vi "Advanced Remez FIR Filter Design.vi"() -> ()   [LabVIEW 2023]
doc: "Demonstrates how to use the DFD Remez Design VI to design advanced finite impulse response (FIR) filters. You can learn how to configure the controls to obtain the ideal filter frequency response of the filter you want to design.\n\nComplete the following steps to use this VI.\n1) Run the VI.\n2) Select one example filter in the <B>Examples</B> list. This VI provides pre-defined filter specifications for each example filter. \n3) View the <B>Specifications</B> page to study the corresponding settings that describe the ideal frequency response.\n4) Observe the plots on the Magnitude Response, Phase Response, and Pole-Zero Plot graphs to see the characteristics of the designed filter.\n5) Compare the <B>Actual Ripples</B> listed on the <B>Magnitude Response</B> page with the <B>ripple constraint</B> specification of each frequency band. Verify if the actual ripples are less than the pre-defined settings.\n6) Click the <B>STOP</B> button to stop this VI."
uses:
  <vilib>/addons/Digital Filter Design/_REMEZ.llb/remez_fir filter type.ctl
  <vilib>/addons/Digital Filter Design/_Objects.llb/DFD Adv Band Spec.ctl
  <vilib>/addons/Digital Filter Design/_Objects.llb/DFD Phase Setting.ctl
  <vilib>/addons/Digital Filter Design/_Objects.llb/DFD Filter Obj.ctl
  <vilib>/addons/Digital Filter Design/_Objects.llb/DFD Filter Coef.ctl
  <vilib>/addons/Digital Filter Design/_Objects.llb/DFD Filter Structure Type Selector.ctl
  <vilib>/addons/Digital Filter Design/_Objects.llb/dfd_Internal Quantization Settings.ctl
  <vilib>/addons/Digital Filter Design/_Objects.llb/dfd_Internal Quantization Srcs.ctl
  <vilib>/addons/Digital Filter Design/_Objects.llb/DFD Coef Norm Type.ctl
  <vilib>/addons/Digital Filter Design/_Objects.llb/DFD Pole-Zero Plot.ctl
  <vilib>/addons/Digital Filter Design/Analysis.llb/DFD Plot Freq Response (Linear-Spaced).vi
  <vilib>/addons/Digital Filter Design/NI_DigFilterLicensed.lvlib
panel:
  in  "filter out":T1={"mSRate_Fs"=1.0, "mSRate_Version"="1.0", "mSRate_Comments"="", "mSRate_OrgCoef"={"type"=enum."Undefined", "gain"=1.0, "coef a (k)"=[], "coef b (v)"=[]}, "mSRate_CurCoef"={"type"=enum."Undefined", "gain"=1.0, "coef a (k)"=[], "coef b (v)"=[]}, "mSRate_Quantized?"=FALSE, "mSRate_QCoef"={"type"=enum."Undefined", "gain"=1.0, "coef a (k)"=[], "coef b (v)"=[]}, "mSRate_QSettings"=[], "mSRate_Order"=0, "mSRate_Scaling"={"mSRate_ScaleByPowerOf2?"=FALSE, "mSRate_ScaleType"=enum."No Norm"}} {"mSRate_QSettings"."source" items=["Coef a/k"=0, "Coef b/v"=7, "Input"=1, "Output"=2, "Multiplicand"=3, "Product"=4, "Sum"=5, "Delay"=6, "Gain"=8]}
  out "Status Str":string="Idle"
  out "Status LED":bool
  in  "Graph":T7(tab)
  out "Actual Ripples":dbl[](array[numeric])
  in  "dB On?":bool
  out "Magnitude Response":cluster{"f0":dbl, "df":dbl, "values":dbl[]}[](graph)
  in  "phase view":T8={"unwrap? (F)"=TRUE, "degree? (F)"=FALSE}
  out "Phase Response":cluster{"f0":dbl, "df":dbl, "values":dbl[]}[](graph)
  out "Z-Plane":T9
  out "Actual Order":i32
  in  "stop":bool
  in  "Selector":enum32{"Examples", "Specifications"}(tab)
  out "Description":string
  in  "Example List":i32(listbox)
  in  "Apply":bool
  in  "Frequencies of Exact Gain [Hz]":dbl[](array[numeric])
  in  "Minimum Order":enum32{"User Defined", "MinEven", "MinOdd"}(ring)
  in  "Band Specifications":T10[](array[typedef])=[{"band specification"=[{"freq"=0.0, "amplitude"=0.0, "weight"=2.0}, {"freq"=0.2, "amplitude"=0.0, "weight"=2.0}], "ripple constraint"=0.0}, {"band specification"=[{"freq"=0.25, "amplitude"=1.0, "weight"=1.0}, {"freq"=0.5, "amplitude"=1.0, "weight"=1.0}], "ripple constraint"=0.0}]
  in  "Sampling Frequency [Hz]":dbl=1.0 format="%.2f"
  in  "Filter Order":i32=52
  in  "Filter Type":T11
  # "Select Help>>Show Context Help and move the cursor over the VI icon for more information."
  # "freq"
  # "amplitude"
  # "weight"
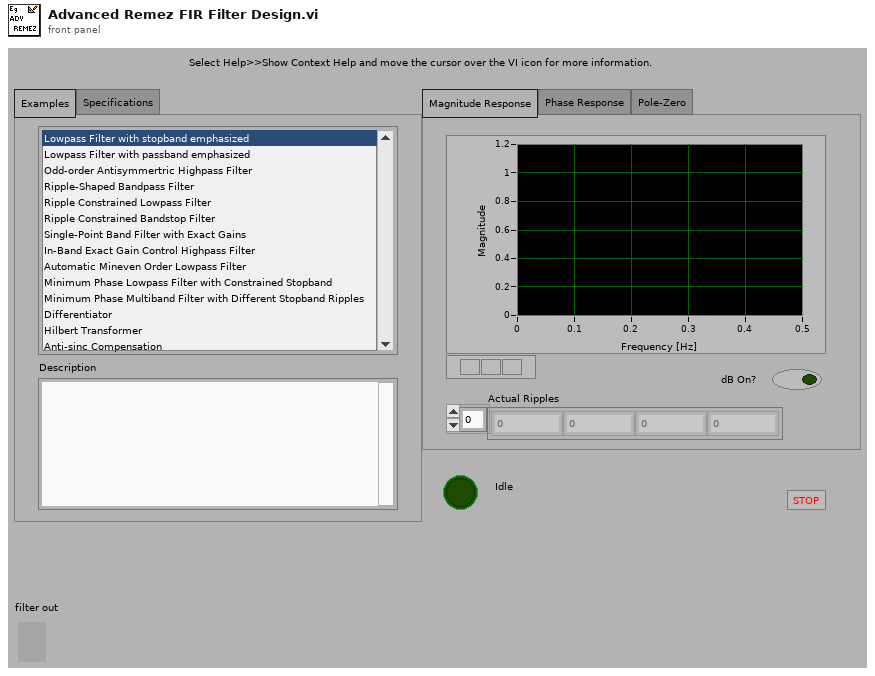
[diagram p1: front panel]
types:
  T1 = typedef "NI_DigFilterLicensed.lvlib/DFD Filter Obj.ctl" = cluster{"mSRate_Fs":dbl, "mSRate_Version":string, "mSRate_Comments":string, "mSRate_OrgCoef":T2, "mSRate_CurCoef":T2, "mSRate_Quantized?":bool, "mSRate_QCoef":T2, "mSRate_QSettings":T4[], "mSRate_Order":i32, "mSRate_Scaling":cluster{"mSRate_ScaleByPowerOf2?":bool, "mSRate_ScaleType":T6}}
  T2 = typedef "NI_DigFilterLicensed.lvlib/DFD Filter Coef.ctl" = cluster{"type":T3, "gain":dbl, "coef a (k)":dbl[], "coef b (v)":dbl[]}
  T3 = typedef "NI_DigFilterLicensed.lvlib/DFD Filter Structure Type Selector.ctl" = enum16{"Undefined", "FIR Direct Form", "FIR Direct Form Transposed", "FIR Symmetric", "FIR Antisymmetric", "IIR Direct Form I", "IIR Direct Form I Transposed", "IIR Direct Form II", "IIR Direct Form II Transposed", "IIR Cascaded Second Order Sections Form I", "IIR Cascaded Second Order Sections Form I Transposed", "IIR Cascaded Second Order Sections Form II", "IIR Cascaded Second Order Sections Form II Transposed", "Lattice Allpass (basic sections)", "Lattice Allpass (one multiplier sections)", "Lattice Allpass (normalized sections)", "Lattice AR (basic sections)", "Lattice AR (one multiplier sections)", "Lattice AR (normalized sections)", "Lattice MA (minimum phase)", "Lattice MA (maximum phase)", "Lattice ARMA (basic sections)", "Lattice ARMA (one multiplier sections)", "Lattice ARMA (normalized sections)"}
  T4 = typedef "NI_DigFilterLicensed.lvlib/dfd_Internal Quantization Settings.ctl" = cluster{"source":T5, "wl":i16, "iwl":i16, "overflow mode":enum16{"Saturation", "Wrap"}, "rounding mode":enum16{"Nearest", "Truncation"}, "signed?":bool}
  T5 = typedef "NI_DigFilterLicensed.lvlib/dfd_Internal Quantization Srcs.ctl" = u16
  T6 = typedef "NI_DigFilterLicensed.lvlib/DFD Coef Norm Type.ctl" = enum16{"No Norm", "Time Domain 1-Norm", "Time Domain 2-Norm", "Time Domain Inf-Norm"}
  T7 = enum32{"Magnitude Response", "Phase Response", "Pole-Zero"}
  T8 = typedef "NI_DigFilterLicensed.lvlib/DFD Phase Setting.ctl" = cluster{"unwrap? (F)":bool, "degree? (F)":bool}
  T9 = typedef "NI_DigFilterLicensed.lvlib/DFD Pole-Zero Plot.ctl" = cluster{dbl[], dbl[]}[]
  T10 = typedef "NI_DigFilterLicensed.lvlib/DFD Adv Band Spec.ctl" = cluster{"band specification":cluster{"freq":dbl, "amplitude":dbl, "weight":dbl}[], "ripple constraint":dbl}
  T11 = typedef "NI_DigFilterLicensed.lvlib/remez_fir filter type.ctl" = enum32{"Symmetric", "Antisymmetric", "Differentiator", "Hilbert", "Minimum Phase", "Maximum Phase"}
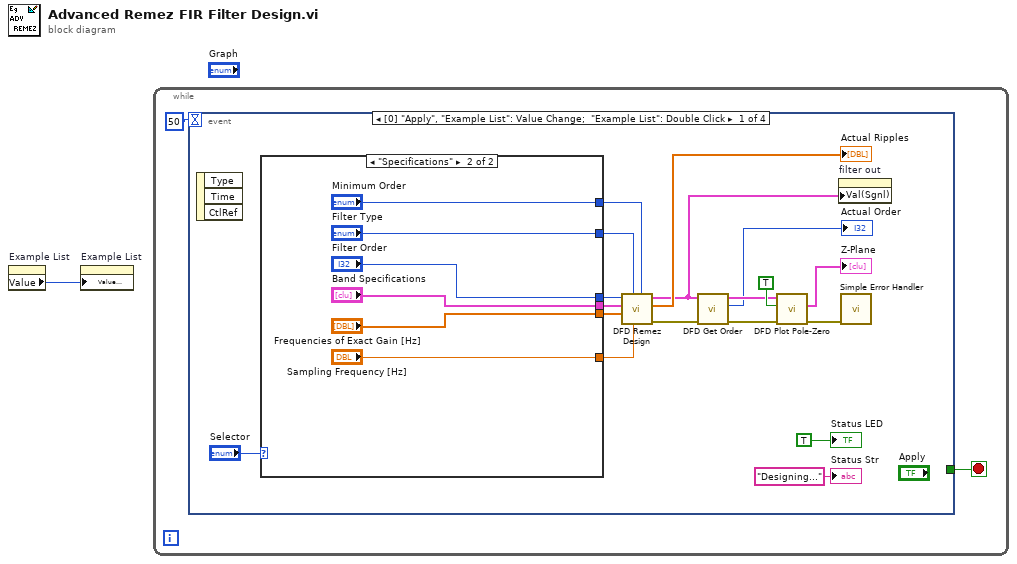
[diagram p0: block diagram]
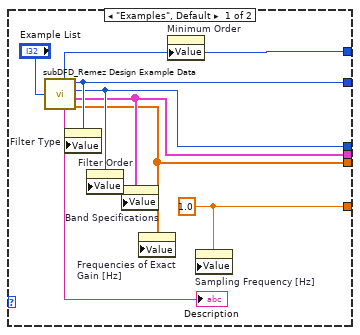
[diagram p2: hidden frame]
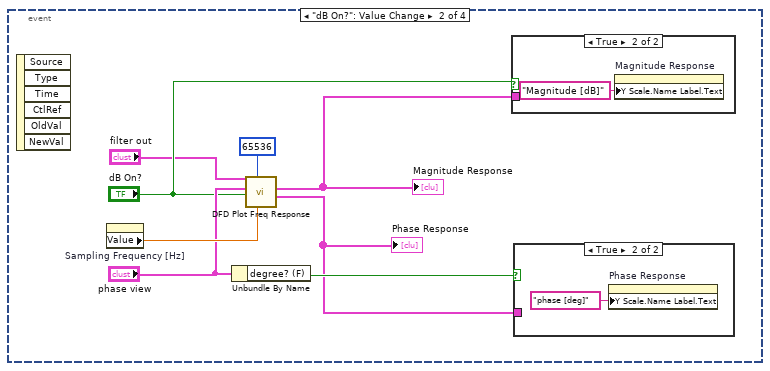
[diagram p3: hidden frame]
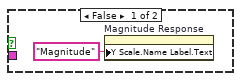
[diagram p4: hidden frame]
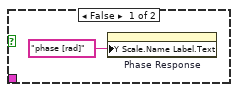
[diagram p5: hidden frame]
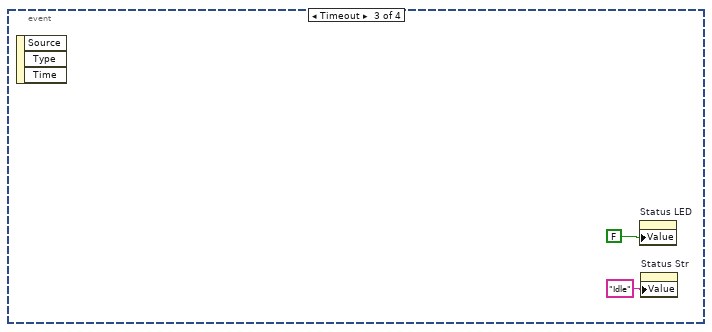
[diagram p6: hidden frame]
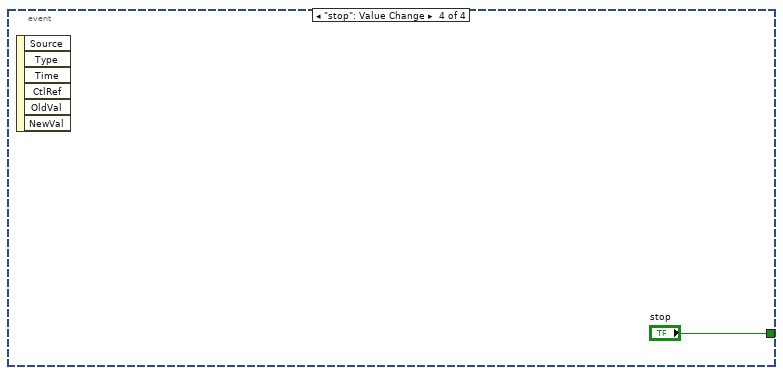
[diagram p7: hidden frame]
diagram:
  n1 = property on="Example List" class="LstBox (strict)"() -> ("Value"=w1:i32)  [unwired: 2 in, 2 out]
  n2 = property on="Example List" class="LstBox (strict)"("Value (Signaling)"=w1) -> ()  [unwired: 2 in, 2 out]
  n3 = while {
    stop <- w3 stop-if-true
    n4 = event shown="[0] \"Apply\", \"Example List\": Value Change;  \"Example List\": Double Click" {
      selector: _ -> [_ _ _ _]
      dyn-events: _ -> [_ _ _ _]
      timeout: 50 -> [_ _ _ _]
      tunnel: [_ _ _ "stop"] -> w3
      event "Apply", "Example List": Value Change; "Example List": Double Click {
        n5 = event-data() -> ()  [unwired: 4 out]
        n6 = case shown="\"Specifications\"" "Selector" {
          tunnel: [w28 "Minimum Order"] -> w18
          tunnel: [w27 "Filter Type"] -> w17
          tunnel: [w26 "Filter Order"] -> w16
          tunnel: [w25 "Band Specifications"] -> w15
          tunnel: [w24 "Frequencies of Exact Gain [Hz]"] -> w14
          tunnel: [w23 "Sampling Frequency [Hz]"] -> w13
          frame "Examples", Default {
            w23 = 1.0 ("fs [Hz]")
            n7 = call "subDFD_Remez Design Example Data.vi"("Example Idx"="Example List") -> ("minimum order"=w28:enum32{"User Defined", "MinEven", "MinOdd"}, "description"=→"Description":string, "phase option"=w27:T11, "order"=w26:i32, "band specs"=w25:T10[], "freqs of exact gain"=w24:dbl[])
            n8 = property on="Filter Type" class="Enum (strict)"("Value"=w27) -> ()  [unwired: 2 in, 2 out]
            n9 = property on="Filter Order" class="DigNum (strict)"("Value"=w26) -> ()  [unwired: 2 in, 2 out]
            n10 = property on="Band Specifications" class="Arr (strict)"("Value"=w25) -> ()  [unwired: 2 in, 2 out]
            n11 = property on="Frequencies of Exact Gain [Hz]" class="Arr (strict)"("Value"=w24) -> ()  [unwired: 2 in, 2 out]
            n12 = property on="Minimum Order" class="Enum (strict)"("Value"=w28) -> ()  [unwired: 2 in, 2 out]
            n13 = property on="Sampling Frequency [Hz]" class="DigNum (strict)"("Value"=w23) -> ()  [unwired: 2 in, 2 out]
          }
          frame "Specifications" {
          }
        }
        n14 = call <vilib>:"DFD Remez Design.vi"("minimum order"=w18, "fs [Hz]"=w13, "filter type"=w17, "freqs of exact gain [Hz]"=w14, "band specs"=w15, "order"=w16) -> ("error out"=w7:errorcluster, "actual ripples"=→"Actual Ripples":dbl[], "filter out"=w8:T1)  [unwired: 1 in, 2 out]
        n15 = call <vilib>:"DFD Get Order.vi"("error in (no error)"=w7, "filter in"=w8) -> ("error out"=w6:errorcluster, "order"=→"Actual Order":i32, "filter out"=w5:T1)  [unwired: 7 in]
        n16 = call <vilib>:"DFD Plot Pole-Zero.vi"("error in (no error)"=w6, "upper half plane only"=TRUE, "filter in"=w5) -> ("error out"=w10:errorcluster, "Z-Plane"=→"Z-Plane":T9)  [unwired: 7 out]
        n17 = property on="filter out" class="Clust (strict)"("Val(Sgnl)"=w8) -> ()  [unwired: 2 in, 2 out]
        n18 = call <vilib>:"Simple Error Handler.vi"("error in (no error)"=w10) -> ()  [unwired: 1 in, 8 out]
        "Status LED" <- TRUE ("Status")
        "Status Str" <- "Designing..." ("String")
      }
      event "dB On?": Value Change {
        n19 = event-data() -> ()  [unwired: 7 out]
        n20 = property on="Sampling Frequency [Hz]" class="DigNum (strict)"() -> ("Value"=w41:dbl)  [unwired: 2 in, 2 out]
        n21 = Unbundle By Name("phase view") -> ("degree? (F)"=w43:bool)
        n22 = call-poly <vilib>:"DFD Plot Freq Response.vi"("fs [Hz]"=w41, "# freq bins"=65536 ("# freq bins (auto)"), "dB on? (T)"="dB On?", "phase view"="phase view", "filter in"="filter out") -> ("phase response"=w40:cluster{"f0":dbl, "df":dbl, "values":dbl[]}[], "magnitude response"=w36:cluster{"f0":dbl, "df":dbl, "values":dbl[]}[])  [unwired: 3 in, 2 out]
        "Magnitude Response" <- w36
        "Phase Response" <- w40
        n23 = case shown="True" "dB On?" {
          tunnel: w36 -> [_ _]
          frame False {
            n24 = property on="Magnitude Response" class="WFGraph (strict)"("Y Scale.Name Label.Text"="Magnitude") -> ()  [unwired: 2 in, 2 out]
          }
          frame True {
            n25 = property on="Magnitude Response" class="WFGraph (strict)"("Y Scale.Name Label.Text"="Magnitude [dB]") -> ()  [unwired: 2 in, 2 out]
          }
        }
        n26 = case shown="True" w43 {
          tunnel: w40 -> [_ _]
          frame False {
            n27 = property on="Phase Response" class="WFGraph (strict)"("Y Scale.Name Label.Text"="phase [rad]") -> ()  [unwired: 2 in, 2 out]
          }
          frame True {
            n28 = property on="Phase Response" class="WFGraph (strict)"("Y Scale.Name Label.Text"="phase [deg]") -> ()  [unwired: 2 in, 2 out]
          }
        }
      }
      event Timeout {
        n29 = event-data() -> ()  [unwired: 4 out]
        n30 = property on="Status LED" class="Bool (strict)"("Value"=FALSE ("Status")) -> ()  [unwired: 2 in, 2 out]
        n31 = property on="Status Str" class="Str"("Value"="Idle" ("Status")) -> ()  [unwired: 2 in, 2 out]
      }
      event "stop": Value Change {
        n32 = event-data() -> ()  [unwired: 7 out]
      }
    }
  }
